vi "Obtain Queue-Live graph data queue interface.vi"(8 "error in (no error)":errorcluster, 11 "Function":enum16{"None", "Release queue"}(ring)) -> (0 "error out":errorcluster, 3 "Live graphs queue":T1)   [LabVIEW 2017]
uses:
  Typedefs/Live graph data queue ref.ctl
  Live graphs queue/Typedefs/Live imaging queue element.ctl
  <vilib>/vision/Image Controls.llb/IMAQ Image.ctl
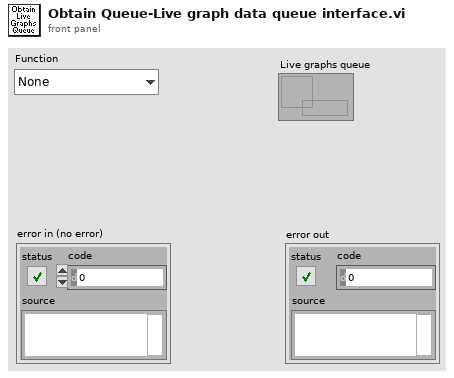
[diagram p1: front panel]
types:
  T1 = typedef "Live graph data queue ref.ctl" = refnum<queue>
  T2 = typedef "Live imaging queue element.ctl" = cluster{"Red channel":T3, "Green channel":T3}
  T3 = typedef "IMAQ Image.ctl" = refnum<image>
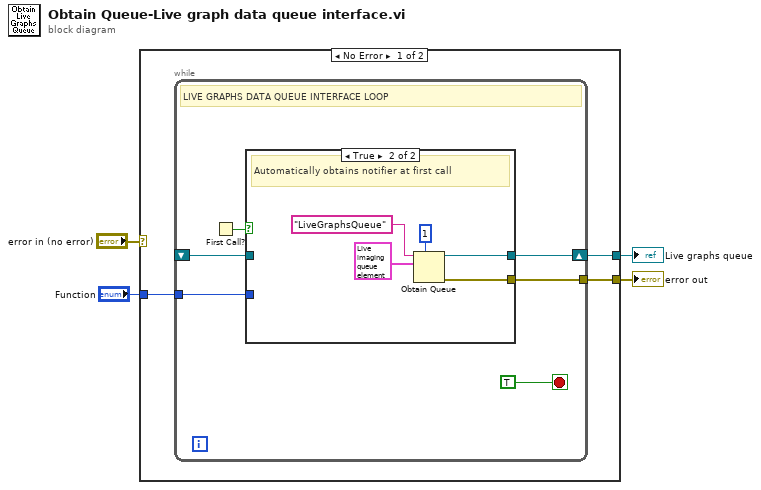
[diagram p0: block diagram]
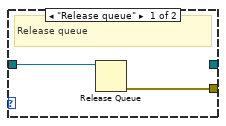
[diagram p3: hidden frame]
diagram:
  n1 = case shown="No Error" "error in (no error)" {
    selector: "error in (no error)" -> [_ w26]
    tunnel: [w7 w26] -> w4
    tunnel: "Function" -> [w6 _]
    tunnel: [w5 _] -> w2
    frame No Error {
      n2 = while {
        tunnel: [w13] -> w7
        tunnel: w6 -> [w11]
        shift-right: [w9] -> w5
        shift-left: _ -> [w8]
        stop <- TRUE stop-if-true
        # "LIVE GRAPHS DATA QUEUE INTERFACE LOOP"
        n3 = First Call?() -> (First Call?: T/F=w10:bool)
        n4 = case shown="True" w10 {
          tunnel: [w16 w25] -> w13
          tunnel: [w14 w24] -> w9
          tunnel: w8 -> [w17 _]
          tunnel: w11 -> [w15 _]
          frame False {
            # "Consecutive calls"
            n5 = case shown="Default" w15 {
              tunnel: w17 -> [w19 w20]
              tunnel: [w18 _] -> w16
              tunnel: [_ w20] -> w14
              frame "Release queue" {
                # "Release queue"
                n6 = Release Queue(queue=w19) -> (error out=w18:errorcluster)  [unwired: 2 in, 2 out]
              }
              frame Default {
                # "None"
              }
            }
          }
          frame True {
            # "Automatically obtains notifier at first call"
            n7 = Obtain Queue(max queue size (-1, unlimited)=1, name (unnamed)="LiveGraphsQueue", element data type=T2 {"Red channel"=refnum, "Green channel"=refnum} ("Element to queue")) -> (queue out=w24:refnum<queue>, error out=w25:errorcluster)  [unwired: 2 in, 1 out]
          }
        }
      }
    }
    frame Error {
    }
  }
  "error out" <- w4
  "Live graphs queue" <- w2
